vi "Konvolucio MCAN120803 Example_0007 Loopback.vi"() -> ()   [LabVIEW 2011]
uses:
  <instrlib>/Konvolucio MCAN120803/Types/MessageType.ctl
  <instrlib>/Konvolucio MCAN120803/Public/Attributes/AttrSetTermination.vi
  <instrlib>/Konvolucio MCAN120803/Public/Attributes/AttrSetLoopback.vi
  <instrlib>/Konvolucio MCAN120803/Public/Attributes/AttrGetRxPendingMsg.vi
  <instrlib>/Konvolucio MCAN120803/Konvolucio MCAN120803.lvlib
panel:
  out "Complete":bool
  out "Timeout":bool
  out "Messages":T1[](array[typedef])
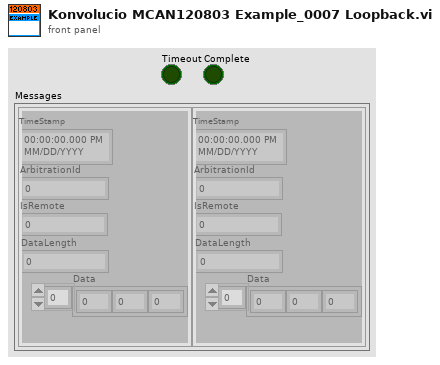
[diagram p1: front panel]
types:
  T1 = typedef "Konvolucio MCAN120803.lvlib/MessageType.ctl" = cluster{"TimeStamp":timestamp, "ArbitrationId":u32, "IsRemote":u8, "DataLength":u8, "Data":u8[]}
  T2 = typedef "Konvolucio MCAN120803.lvlib/CanHandleType.ctl" = cluster{"AdapterDevice":refnum<k24>}
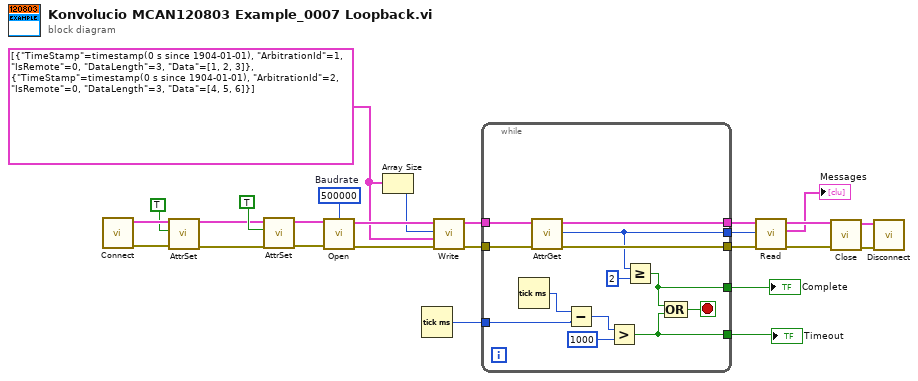
[diagram p0: block diagram]
diagram:
  w15 = T1[] [{"TimeStamp"=timestamp(0 s since 1904-01-01), "ArbitrationId"=1, "IsRemote"=0, "DataLength"=3, "Data"=[1, 2, 3]}, {"TimeStamp"=timestamp(0 s since 1904-01-01), "ArbitrationId"=2, "IsRemote"=0, "DataLength"=3, "Data"=[4, 5, 6]}] ("Messages")
  w26 = u32 500000  # Baudrate
  n1 = call <instrlib>:"Connect.vi"() -> ("error out"=w25:errorcluster, "CanHandleOut"=w24:T2)  [unwired: 10 in]
  n2 = call-poly <instrlib>:"AttrSet.vi"("error in"=w25, "Enabled"=TRUE, "CanHandleIn"=w24) -> ("error out"=w8:errorcluster, "CanHandleOut"=w5:T2)  [unwired: 6 in]
  n3 = call-poly <instrlib>:"AttrSet.vi"("error in"=w8, "Enabled"=TRUE, "CanHandleIn"=w5) -> ("error out"=w7:errorcluster, "CanHandleOut"=w4:T2)  [unwired: 6 in]
  n4 = call <instrlib>:"Open.vi"("error in"=w7, "Baudrate"=w26, "CanHandleIn"=w4) -> ("error out"=w16:errorcluster, "CanHandleOut"=w17:T2)  [unwired: 7 in]
  n5 = Array Size(array=w15) -> (size(s)=w14:i32)
  n6 = Tick Count (ms)() -> (millisecond timer value=w11:u32)
  n7 = call <instrlib>:"Write.vi"("error in"=w16, "Messages"=w15, "Number to Write"=w14, "CanHandleIn"=w17) -> ("error out"=w13:errorcluster, "CanHandleOut"=w12:T2)  [unwired: 4 in]
  n8 = while {
    tunnel: w13 -> [w39]
    tunnel: w12 -> [w38]
    tunnel: w11 -> [w37]
    tunnel: [w33] -> w10
    tunnel: [w32] -> w9
    tunnel: [w29] -> w3
    tunnel: [w28] -> w2
    tunnel: [w27] -> w1
    stop <- w30 stop-if-true
    n9 = Tick Count (ms)() -> (millisecond timer value=w36:u32)
    n10 = call-poly <instrlib>:"AttrGet.vi"("error in"=w39, "CanHandleIn"=w38) -> ("error out"=w33:errorcluster, "Value"=w27:i32, "CanHandleOut"=w32:T2)  [unwired: 7 in]
    n11 = Subtract(x=w36, y=w37) -> (x-y=w35:u32)
    n12 = Greater?(x=w35, y=u32 1000) -> (0:w29:bool)
    n13 = Greater Or Equal?(x=w27, y=2) -> (x >= y?=w28:bool)
    n14 = Compound Arithmetic op=OR(w28, w29) -> (w30:bool)
  }
  "Timeout" <- w3
  "Complete" <- w2
  n15 = call <instrlib>:"Read.vi"("error in"=w10, "Request Number of Message"=w1, "CanHandleIn"=w9) -> ("error out"=w20:errorcluster, "Messages"=→"Messages":T1[], "CanHandleOut"=w19:T2)  [unwired: 6 in]
  n16 = call <instrlib>:"Close.vi"("error in"=w20, "CanHandleIn"=w19) -> ("error out"=w22:errorcluster, "CanHandleOut"=w21:T2)  [unwired: 8 in]
  n17 = call <instrlib>:"Disconnect.vi"("error in"=w22, "CanHandleIn"=w21) -> ()  [unwired: 9 in, 1 out]
